vi "ResizeHistory.vi"(11 "State In":T1 caption="State") -> (3 "State Out":T1 caption="State")   [LabVIEW 2009, in "HistoryPath.xctl"]
uses:
  HistoryPath.xctl
  State.ctl
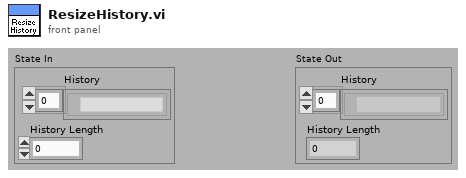
[diagram p1: front panel]
types:
  T1 = typedef "HistoryPath.xctl/State.ctl" = cluster{"History":path[], "History Length":i32}
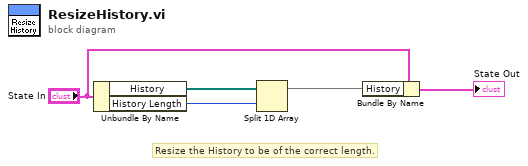
[diagram p0: block diagram]
diagram:
  # "Resize the History to be of the correct length."
  n1 = Unbundle By Name("State In") -> ("History"=w5:path[], "History Length"=w4:i32)
  n2 = Split 1D Array(array=w5, index=w4) -> (first subarray=w1:path[])  [unwired: 1 out]
  n3 = Bundle By Name(cluster="State In", "History"=w1) -> (→"State Out":T1)
